vi "Set Package BuildSpec MinVersion Dependency.vi"(5 "dependency package name":string, 7 "version":string, 8 "error in (no error)":errorcluster, 10 "package buildspec ref in":refnum<vi>, 11 "project ref in":refnum<vi>) -> (0 "error out":errorcluster, 1 "version updated?":bool, 2 "package buildspec ref out":refnum<vi>, 3 "project ref out":refnum<vi>)   [LabVIEW 2018, in "NIPKG BuildSpec API.lvlib"]
doc: "This VI sets the version of the specified dependency package in the Package build specification of a LabVIEW project.\n\nNote: To persist the updated version in the LabVIEW project file, you must Save the project after this VI finishes executing."
uses:
  NIPKG BuildSpec API.lvlib
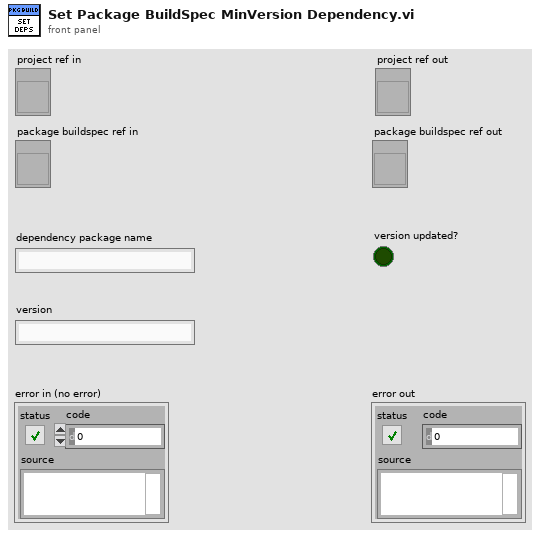
[diagram p1: front panel]
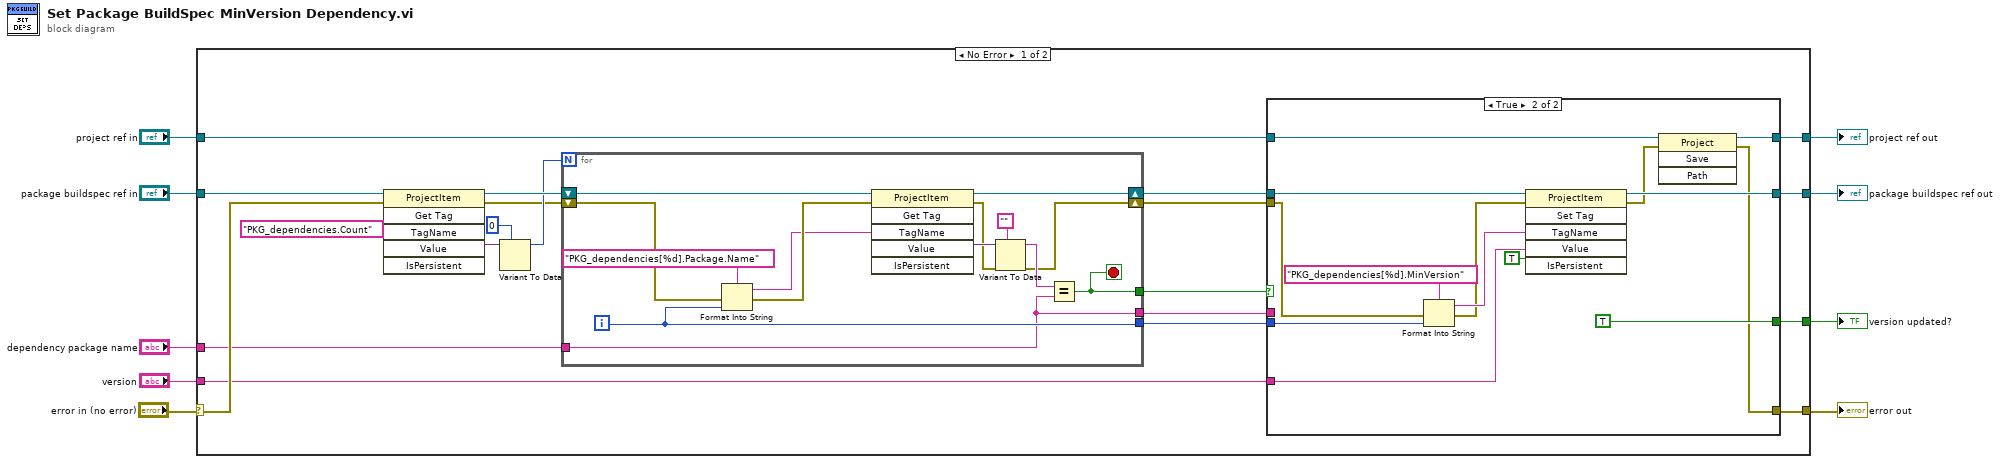
[diagram p0: block diagram]
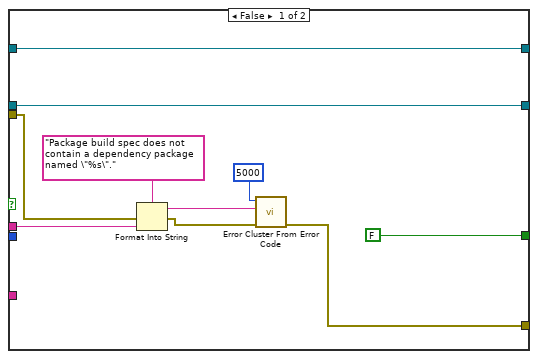
[diagram p2: hidden frame]
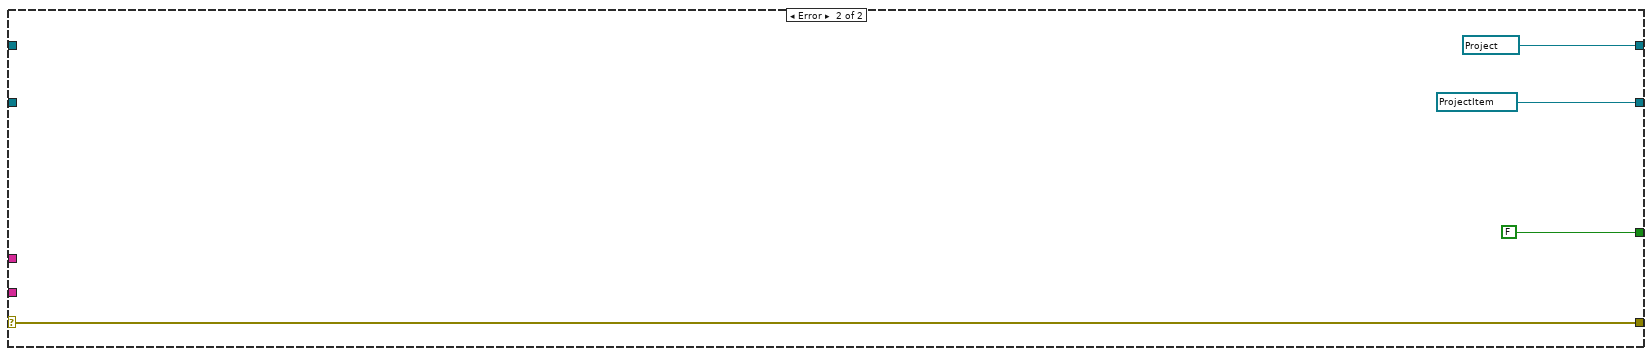
[diagram p3: hidden frame]
diagram:
  n1 = case shown="No Error" "error in (no error)" {
    selector: "error in (no error)" -> [w23 w71]
    tunnel: "package buildspec ref in" -> [w24 _]
    tunnel: "dependency package name" -> [w21 _]
    tunnel: "version" -> [w16 _]
    tunnel: [w14 w71] -> w5
    tunnel: [w13 refnum<vi> refnum ("package buildspec ref in")] -> w4
    tunnel: [w12 FALSE] -> w3
    tunnel: "project ref in" -> [w11 _]
    tunnel: [w10 refnum<vi> refnum ("project ref in")] -> w1
    frame No Error {
      n2 = invoke class="ProjectItem" method="Get Tag"(reference=w24, error in=w23, "TagName"="PKG_dependencies.Count" ("Tag Name")) -> (reference out=w26:refnum<vi>, error out=w22:errorcluster, "Value"=w28:variant)  [unwired: 3 in, 3 out]
      n3 = Variant To Data(type=0, Variant=w28) -> (data=w25:i32)  [unwired: 1 in, 1 out]
      n4 = for {
        N: w25 -> [_]
        shift-right: [w56] -> w18
        shift-left: w22 -> [w63]
        tunnel: w21 -> [w54]
        tunnel: [w61] -> w20
        shift-right: [w60] -> w17
        shift-left: w26 -> [w65]
        tunnel: [w58] -> w19
        tunnel: [w54] -> w15
        i -> [w58]
        stop <- w61 stop-if-true
        n5 = Format Into String(format string="PKG_dependencies[%d].Package.Name", error in=w63, w58) -> (resulting string=w55:string, error out=w59:errorcluster)  [unwired: 1 in]
        n6 = invoke class="ProjectItem" method="Get Tag"(reference=w65, error in=w59, "TagName"=w55) -> (reference out=w60:refnum<vi>, error out=w57:errorcluster, "Value"=w67:variant)  [unwired: 3 in, 3 out]
        n7 = Variant To Data(error in=w57, type="", Variant=w67) -> (data=w62:string, error out=w56:errorcluster)
        n8 = Equal?(x=w62, y=w54) -> (x = y?=w61:bool)
      }
      n9 = case shown="True" w20 {
        tunnel: w19 -> [_ w53]
        tunnel: w18 -> [w34 w51]
        tunnel: w17 -> [w39 w50]
        tunnel: w16 -> [_ w48]
        tunnel: [w39 w46] -> w13
        tunnel: w15 -> [w36 _]
        tunnel: [w32 w42] -> w14
        tunnel: [FALSE TRUE] -> w12
        tunnel: w11 -> [w30 w41]
        tunnel: [w30 w40] -> w10
        frame False {
          n10 = Format Into String(format string="Package build spec does not contain a dependency package named \"%s\"." ("error message (\"\")"), error in=w34, w36) -> (resulting string=w35:string, error out=w33:errorcluster)  [unwired: 1 in]
          n11 = call <vilib>:"Error Cluster From Error Code.vi"("error in (no error)"=w33, "error message (\"\")"=w35, "error code (0)"=5000) -> ("error out"=w32:errorcluster)  [unwired: 6 in]
        }
        frame True {
          n12 = Format Into String(format string="PKG_dependencies[%d].MinVersion", error in=w51, w53) -> (resulting string=w49:string, error out=w45:errorcluster)  [unwired: 1 in]
          n13 = invoke class="ProjectItem" method="Set Tag"(reference=w50, error in=w45, "TagName"=w49, "Value"=w48, "IsPersistent"=TRUE ("Is Persistent")) -> (reference out=w46:refnum<vi>, error out=w43:errorcluster)  [unwired: 1 in, 4 out]
          n14 = invoke class="Project" method="Save"(reference=w41, error in=w43) -> (reference out=w40:refnum<vi>, error out=w42:errorcluster)  [unwired: 2 in, 2 out]
        }
      }
    }
    frame Error {
    }
  }
  "error out" <- w5
  "package buildspec ref out" <- w4
  "version updated?" <- w3
  "project ref out" <- w1
